vi "elevator task.vi"() -> ()   [LabVIEW 2016, in "elevator.lvlib"]
uses:
  elevator.lvlib
panel:
  in  "停止":bool
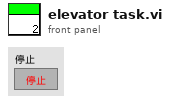
[diagram p1: front panel]
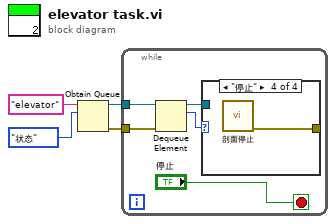
[diagram p0: block diagram]
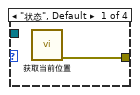
[diagram p2: hidden frame]
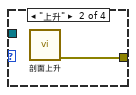
[diagram p3: hidden frame]
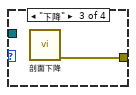
[diagram p4: hidden frame]
diagram:
  n1 = Obtain Queue(name (unnamed)="elevator" ("名称（未命名）"), element data type=enum16{"状态", "上升", "下降", "停止"}."状态" ("枚举")) -> (queue out=w2:refnum<queue>, error out=w1:errorcluster)  [unwired: 3 in, 1 out]
  n2 = while {
    tunnel: w2 -> [w8]
    tunnel: w1 -> [w9]
    stop <- "停止" stop-if-true
    n3 = Dequeue Element(queue=w8, error in (no error)=w9) -> (queue out=w6:refnum<queue>, element=w7:enum16{"状态", "上升", "下降", "停止"})  [unwired: 1 in, 2 out]
    n4 = case shown="\"停止\"" w7 {
      tunnel: w6 -> [_ _ _ _]
      tunnel: [w10 w11 w12 w13] -> _
      frame "状态", Default {
        n5 = call "获取当前位置.vi"() -> ("error out"=w10:errorcluster)  [unwired: 9 in, 2 out]
      }
      frame "上升" {
        n6 = call "剖面上升.vi"() -> ("error out"=w11:errorcluster)  [unwired: 11 in]
      }
      frame "下降" {
        n7 = call "剖面下降.vi"() -> ("error out"=w12:errorcluster)  [unwired: 11 in]
      }
      frame "停止" {
        n8 = call "剖面停止.vi"() -> ("error out"=w13:errorcluster)  [unwired: 11 in]
      }
    }
  }
